vi "Teleop.vi"(10 "Match Info":T1={"Autonomous Elapsed Seconds"=0.0, "TeleOp Elapsed Seconds"=0.0, "Disabled Elapsed Seconds"=0.0, "Visited Autonomous"=FALSE, "Visited TeleOp"=FALSE, "Visited Disabled"=FALSE, "Autonomous Settings"={"Autonomous Style"=enum."Independent", "VI Refnum"=refnum}}, 11 "Call Context":T2) -> ()   [LabVIEW 2017]
doc: "This VI is called for each TeleOp packet received from the DS where the robot is not disabled. It is often used to read from the joysticks and update I/O or to update setpoints for timed control loops. It should complete and return within 20 milliseconds or it may miss DS packets."
uses:
  <vilib>/Rock Robotics/WPI/DriverStation/WPI_DriverStationDerivedRobotMode.ctl
  <vilib>/Rock Robotics/WPI/DriverStation/WPI_DriverStationMatch Info.ctl
  <vilib>/Rock Robotics/Network Tables/NT Read Boolean.vi
  <vilib>/Rock Robotics/Network Tables/NT Read Number.vi
  <vilib>/Rock Robotics/WPI/Utilities/WPI_GetSetVariantRefNum.vi
  <vilib>/Rock Robotics/Network Tables/NT Write Boolean Array.vi
  <vilib>/Rock Robotics/Network Tables/NT Write Numeric Array.vi
  Robot Global Data.vi
panel:
  out "Sample Slider 0":dbl(slide) scale=0.0..5.0
  out "Sample Boolean 1":bool
  out "Sample Boolean 0":bool
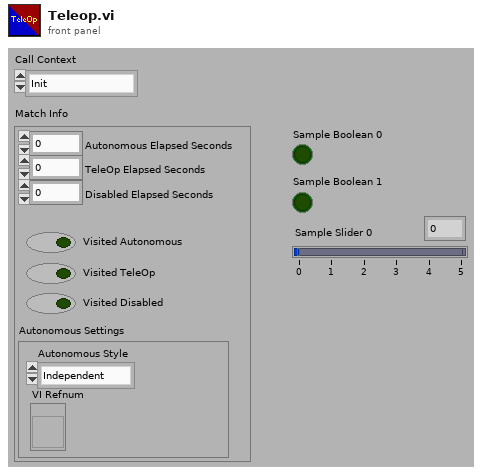
[diagram p1: front panel]
types:
  T1 = typedef "WPI_DriverStationMatch Info.ctl" = cluster{"Autonomous Elapsed Seconds":dbl, "TeleOp Elapsed Seconds":dbl, "Disabled Elapsed Seconds":dbl, "Visited Autonomous":bool, "Visited TeleOp":bool, "Visited Disabled":bool, "Autonomous Settings":cluster{"Autonomous Style":enum16{"Iterative", "Independent"}, "VI Refnum":refnum<vi>}}
  T2 = typedef "WPI_DriverStationDerivedRobotMode.ctl" = enum16{"Init", "Execute", "Stop"}
  T3 = typedef "WPI_JoystickDevRef.ctl" = cluster{"Device":T4}
  T4 = typedef "WPI_JoystickDeviceEnum.ctl" = enum16{"USB 0", "USB 1", "USB 2", "USB 3", "USB 4", "USB 5"}
  T5 = cluster{"Axes[0]":dbl, "Axes[1]":dbl, "Axes[2]":dbl, "Axes[3]":dbl, "Axes[4]":dbl, "Axes[5]":dbl, "Axes[6]":dbl, "Axes[7]":dbl, "Axes[8]":dbl}
  T6 = cluster{"Buttons[0]":bool, "Buttons[1]":bool, "Buttons[2]":bool, "Buttons[3]":bool, "Buttons[4]":bool, "Buttons[5]":bool, "Buttons[6]":bool, "Buttons[7]":bool, "Buttons[8]":bool}
  T7 = enum16{"SingleJoystick", "DoubleJoystick", "GameController"}
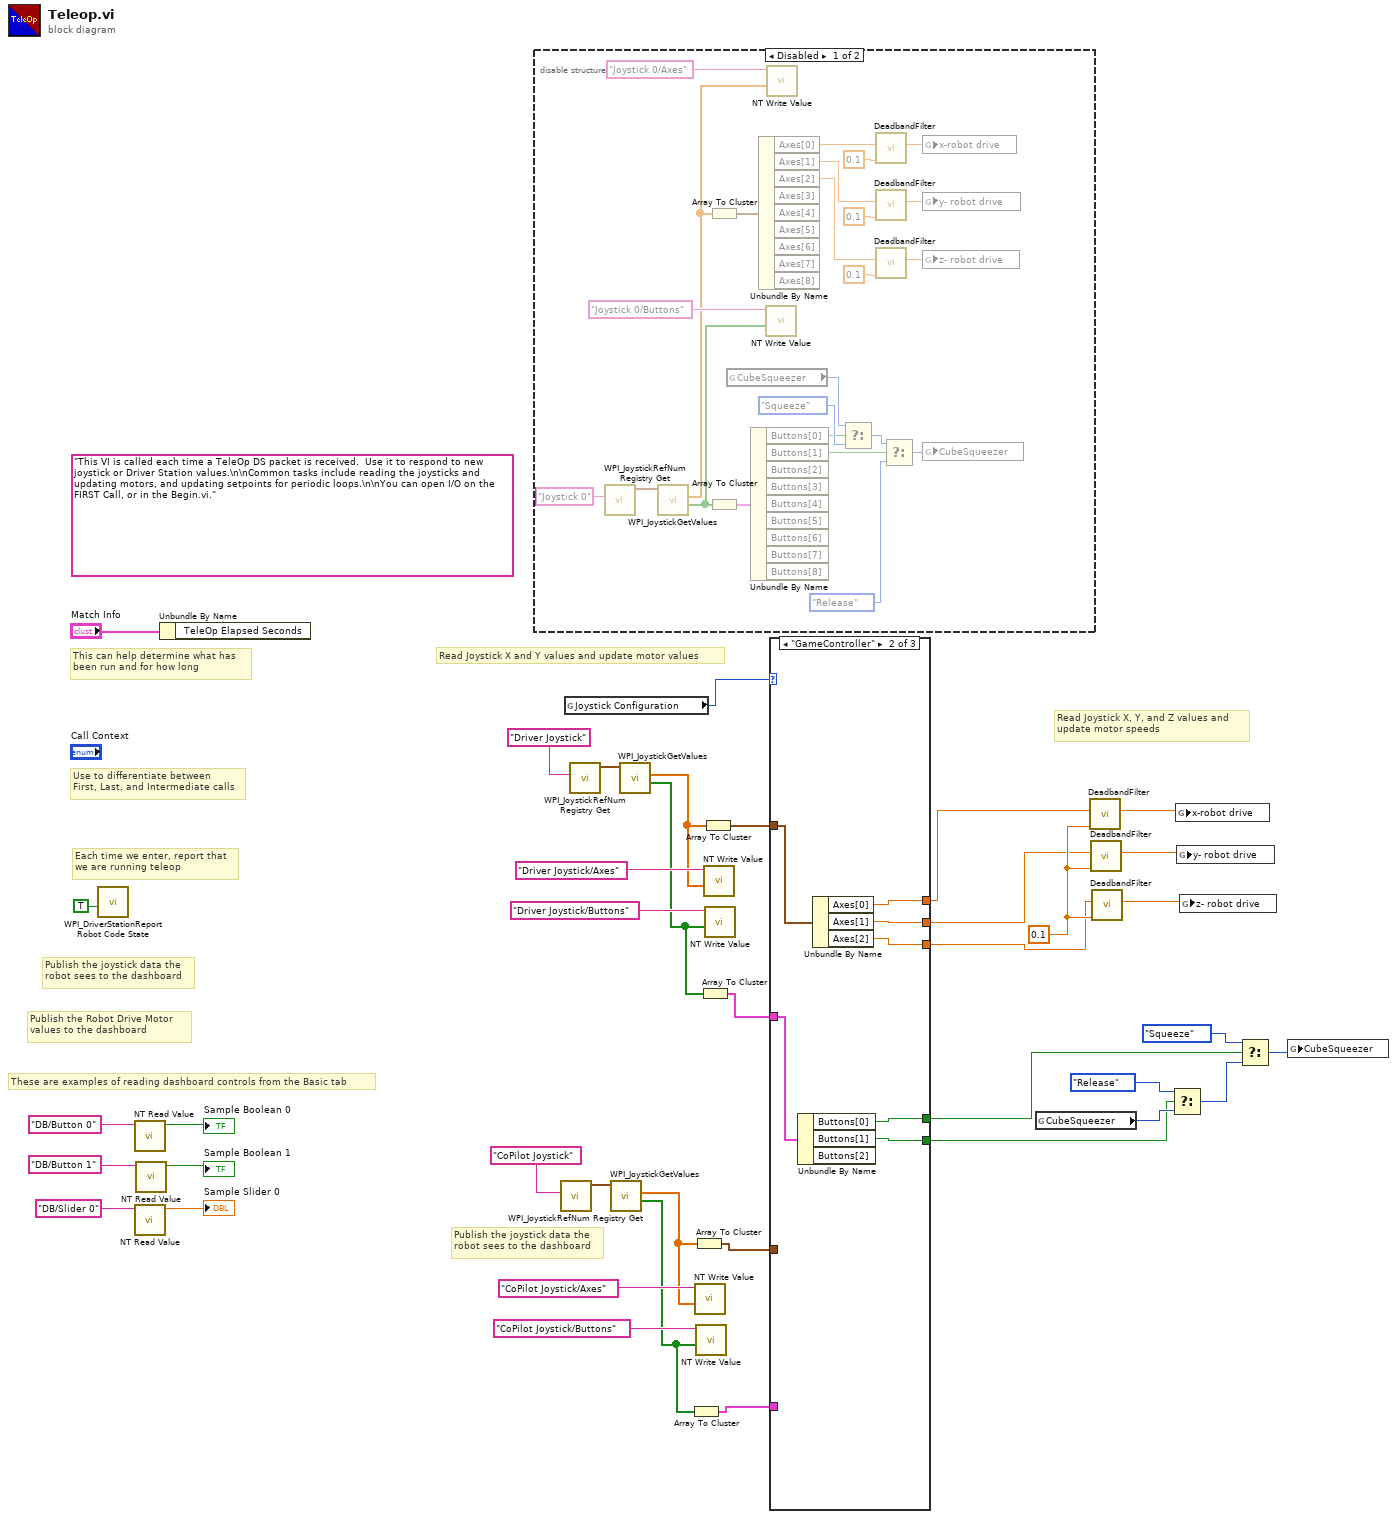
[diagram p0: block diagram]
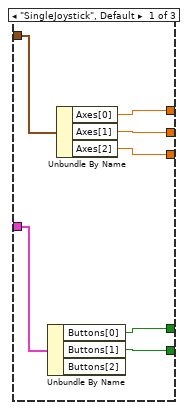
[diagram p2: hidden frame]
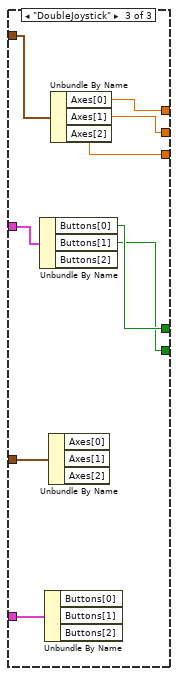
[diagram p3: hidden frame]
diagram:
  w22 = 0.1 ("guardband value")
  (unwired) "This VI is called each time a TeleOp DS packet is received.  Use it to respond to new joystick or Driver Station values.\n\nCommon tasks include reading the joysticks and updating motors, and updating setpoints for periodic loops.\n\nYou can open I/O on the FIRST Call, or in the Begin.vi."
  # "Publish the joystick data the\nrobot sees to the dashboard"
  # "Read Joystick X, Y, and Z values and \nupdate motor speeds"
  # "These are examples of reading dashboard controls from the Basic tab"
  # "Publish the Robot Drive Motor\nvalues to the dashboard"
  # "Publish the joystick data the\nrobot sees to the dashboard"
  # "Each time we enter, report that\nwe are running teleop"
  # "Use to differentiate between\nFirst, Last, and Intermediate calls"
  # "This can help determine what has\nbeen run and for how long"
  # "Read Joystick X and Y values and update motor values"
  n1 = call <vilib>:"WPI_DriverStationReport Robot Code State.vi"("TeleOp"=TRUE ("Autonomous")) -> ()  [unwired: 10 in, 1 out]
  n2 = call-poly <vilib>:"NT Read Value.vi"("Name"="DB/Button 0" ("refnum name")) -> ("Boolean"=→"Sample Boolean 0":bool)  [unwired: 9 in, 1 out]
  n3 = call-poly <vilib>:"NT Read Value.vi"("Name"="DB/Slider 0" ("refnum name")) -> ("Numeric"=→"Sample Slider 0":dbl)  [unwired: 9 in, 1 out]
  n4 = call-poly <vilib>:"NT Read Value.vi"("Name"="DB/Button 1" ("refnum name")) -> ("Boolean"=→"Sample Boolean 1":bool)  [unwired: 9 in, 1 out]
  n5 = Unbundle By Name("Match Info") -> ()  [unwired: 1 out]
  n6 = disable-structure shown="Disabled" {
    frame Disabled {
      n7 = call <vilib>:"WPI_JoystickRefNum Registry Get.vi"("refnum name"="Joystick 0") -> ("JoystickDevRef"=w62:T3)  [unwired: 1 in, 9 out]
      n8 = call <vilib>:"WPI_JoystickGetValues.vi"("JoystickDevRef"=w62) -> ("Buttons"=w57:bool[], "Axes"=w59:dbl[])  [unwired: 6 in, 3 out]
      n9 = Array To Cluster(array=w59) -> (cluster=w58:T5)
      n10 = Array To Cluster(array=w57) -> (cluster=w56:T6)
      n11 = global read "Robot Global Data.vi" "CubeSqueezer"() -> (w47:enum16{"Squeeze", "Release"})
      n12 = Unbundle By Name(w56) -> ("Buttons[0]"=w41:bool, "Buttons[1]"=w40:bool)  [unwired: 7 out]
      n13 = Unbundle By Name(w58) -> ("Axes[0]"=w42:dbl, "Axes[1]"=w43:dbl, "Axes[2]"=w44:dbl)  [unwired: 6 out]
      n14 = call-poly <vilib>:"NT Write Value.vi"("Boolean Array"=w57, "Name"="Joystick 0/Buttons") -> ()  [unwired: 9 in, 1 out]
      n15 = call-poly <vilib>:"NT Write Value.vi"("Numeric Array"=w59, "Name"="Joystick 0/Axes") -> ()  [unwired: 9 in, 1 out]
      n16 = Select(t=w47, s=w41, f=enum16{"Squeeze", "Release"}."Squeeze" ("CubeSqueezer")) -> (s? t:f=w46:enum16{"Squeeze", "Release"})
      n17 = call "DeadbandFilter.vi"("guardband value"=0.1, "JoystickAxis"=w42) -> ("FilteredJoystickAxis"=w55:dbl)  [unwired: 9 in]
      n18 = call "DeadbandFilter.vi"("guardband value"=0.1, "JoystickAxis"=w43) -> ("FilteredJoystickAxis"=w53:dbl)  [unwired: 9 in]
      n19 = call "DeadbandFilter.vi"("guardband value"=0.1, "JoystickAxis"=w44) -> ("FilteredJoystickAxis"=w51:dbl)  [unwired: 9 in]
      n20 = Select(t=w46, s=w40, f=enum16{"Squeeze", "Release"}."Release" ("CubeSqueezer")) -> (s? t:f=w45:enum16{"Squeeze", "Release"})
      n21 = global write "Robot Global Data.vi" "x-robot drive"(w55) -> ()
      n22 = global write "Robot Global Data.vi" "y- robot drive"(w53) -> ()
      n23 = global write "Robot Global Data.vi" "z- robot drive"(w51) -> ()
      n24 = global write "Robot Global Data.vi" "CubeSqueezer"(w45) -> ()
    }
    frame Enabled {
    }
  }
  n25 = call <vilib>:"WPI_JoystickRefNum Registry Get.vi"("refnum name"="CoPilot Joystick") -> ("JoystickDevRef"=w15:T3)  [unwired: 1 in, 9 out]
  n26 = global read "Robot Global Data.vi" "Joystick Configuration"() -> (w10:T7)
  n27 = call <vilib>:"WPI_JoystickRefNum Registry Get.vi"("refnum name"="Driver Joystick") -> ("JoystickDevRef"=w30:T3)  [unwired: 1 in, 9 out]
  n28 = call <vilib>:"WPI_JoystickGetValues.vi"("JoystickDevRef"=w15) -> ("Buttons"=w11:bool[], "Axes"=w12:dbl[])  [unwired: 6 in, 3 out]
  n29 = call <vilib>:"WPI_JoystickGetValues.vi"("JoystickDevRef"=w30) -> ("Buttons"=w26:bool[], "Axes"=w27:dbl[])  [unwired: 6 in, 3 out]
  n30 = Array To Cluster(array=w11) -> (cluster=w4:T6)
  n31 = Array To Cluster(array=w12) -> (cluster=w5:T5)
  n32 = call-poly <vilib>:"NT Write Value.vi"("Numeric Array"=w12, "Name"="CoPilot Joystick/Axes") -> ()  [unwired: 9 in, 1 out]
  n33 = call-poly <vilib>:"NT Write Value.vi"("Boolean Array"=w11, "Name"="CoPilot Joystick/Buttons") -> ()  [unwired: 9 in, 1 out]
  n34 = Array To Cluster(array=w26) -> (cluster=w3:T6)
  n35 = Array To Cluster(array=w27) -> (cluster=w9:T5)
  n36 = call-poly <vilib>:"NT Write Value.vi"("Numeric Array"=w27, "Name"="Driver Joystick/Axes") -> ()  [unwired: 9 in, 1 out]
  n37 = call-poly <vilib>:"NT Write Value.vi"("Boolean Array"=w26, "Name"="Driver Joystick/Buttons") -> ()  [unwired: 9 in, 1 out]
  n38 = case shown="\"GameController\"" w10 {
    tunnel: [w70 w77 w85] -> w8
    tunnel: [w69 w76 w84] -> w7
    tunnel: [w68 w75 w83] -> w6
    tunnel: [w67 w74 w79] -> w2
    tunnel: [w66 w73 w78] -> w1
    tunnel: w9 -> [w65 w72 w86]
    tunnel: w5 -> [_ _ w82]
    tunnel: w4 -> [_ _ w81]
    tunnel: w3 -> [w64 w71 w80]
    frame "SingleJoystick", Default {
      n39 = Unbundle By Name(w64) -> ("Buttons[0]"=w67:bool, "Buttons[1]"=w66:bool)  [unwired: 1 out]
      n40 = Unbundle By Name(w65) -> ("Axes[0]"=w70:dbl, "Axes[1]"=w69:dbl, "Axes[2]"=w68:dbl)
    }
    frame "GameController" {
      n41 = Unbundle By Name(w71) -> ("Buttons[0]"=w74:bool, "Buttons[1]"=w73:bool)  [unwired: 1 out]
      n42 = Unbundle By Name(w72) -> ("Axes[0]"=w77:dbl, "Axes[1]"=w76:dbl, "Axes[2]"=w75:dbl)
    }
    frame "DoubleJoystick" {
      n43 = Unbundle By Name(w80) -> ("Buttons[0]"=w79:bool, "Buttons[1]"=w78:bool)  [unwired: 1 out]
      n44 = Unbundle By Name(w81) -> ()  [unwired: 3 out]
      n45 = Unbundle By Name(w82) -> ()  [unwired: 3 out]
      n46 = Unbundle By Name(w86) -> ("Axes[0]"=w85:dbl, "Axes[1]"=w84:dbl, "Axes[2]"=w83:dbl)
    }
  }
  n47 = global read "Robot Global Data.vi" "CubeSqueezer"() -> (w21:enum16{"Squeeze", "Release"})
  n48 = call "DeadbandFilter.vi"("guardband value"=w22, "JoystickAxis"=w8) -> ("FilteredJoystickAxis"=w25:dbl)  [unwired: 9 in]
  n49 = call "DeadbandFilter.vi"("guardband value"=w22, "JoystickAxis"=w7) -> ("FilteredJoystickAxis"=w24:dbl)  [unwired: 9 in]
  n50 = call "DeadbandFilter.vi"("guardband value"=w22, "JoystickAxis"=w6) -> ("FilteredJoystickAxis"=w23:dbl)  [unwired: 9 in]
  n51 = Select(t=enum16{"Squeeze", "Release"}."Release" ("CubeSqueezer"), s=w1, f=w21) -> (s? t:f=w17:enum16{"Squeeze", "Release"})
  n52 = global write "Robot Global Data.vi" "x-robot drive"(w25) -> ()
  n53 = global write "Robot Global Data.vi" "y- robot drive"(w24) -> ()
  n54 = global write "Robot Global Data.vi" "z- robot drive"(w23) -> ()
  n55 = Select(t=enum16{"Squeeze", "Release"}."Squeeze" ("CubeSqueezer"), s=w2, f=w17) -> (s? t:f=w18:enum16{"Squeeze", "Release"})
  n56 = global write "Robot Global Data.vi" "CubeSqueezer"(w18) -> ()
